vi "select_initial.vi"(9 "Column name":string="fcode_full", 10 "Column table":string[](array[string]), 11 "table":string) -> (2 "Data to write":bool, 3 "parameters":string)   [LabVIEW 2019, in "PostgreSQL.lvlib"]
uses:
  PostgreSQL.lvlib
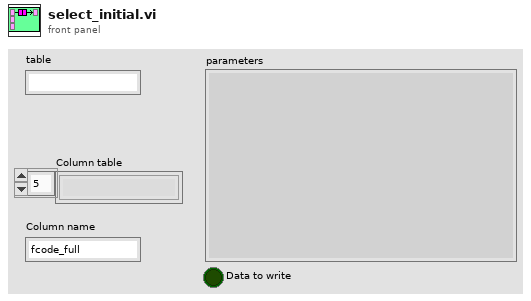
[diagram p1: front panel]
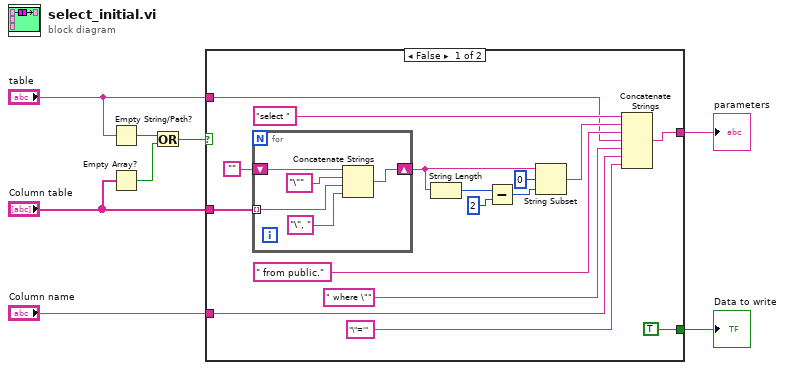
[diagram p0: block diagram]
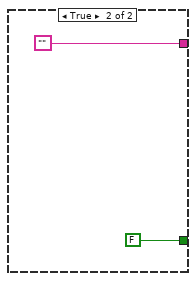
[diagram p2: hidden frame]
diagram:
  n1 = Empty String/Path?(string/path="table") -> (empty?=w5:bool)
  n2 = Empty Array?(array="Column table") -> (empty?=w4:bool)
  n3 = Or(x=w5, y=w4) -> (x .or. y?=w3:bool)
  n4 = case shown="False" w3 {
    tunnel: [w14 ""] -> w8
    tunnel: "table" -> [w13 _]
    tunnel: "Column table" -> [w12 _]
    tunnel: [TRUE FALSE] -> w2
    tunnel: "Column name" -> [w9 _]
    frame False {
      n5 = for {
        shift-right: [w27] -> w23
        shift-left: "" -> [w25]
        tunnel: w12 -> [w26] mode=indexing
        n6 = Concatenate Strings(w25, "\"" ("table"), w26, "\", " ("table")) -> (w27:string)
      }
      n7 = String Length(string=w23) -> (length=w22:i32)
      n8 = Subtract(x=w22, y=2) -> (x-y=w17:i32)
      n9 = String Subset(string=w23, offset (0)=0, length (rest)=w17) -> (substring=w20:string)
      n10 = Concatenate Strings("select " ("table"), w20, " from public." ("table"), w13, " where \"" ("string"), w9, "\"='" ("string")) -> (w14:string)
    }
    frame True {
    }
  }
  "parameters" <- w8
  "Data to write" <- w2
